vi "Pick or Place Part.vi"(5 "Part Vacuum Line":string, 6 "Pick or Place":enum16{"Pick", "Place"}(ring), 7 "Part Named Position":string, 8 "error in (no error)":errorcluster, 9 "Part Rotation":dbl, 10 "Part Position":refnum<class "Vec3d.lvclass">, 11 "Gantry in":refnum<class "Gantry.lvclass">) -> (0 "error out":errorcluster, 3 "Gantry out":refnum<class "Gantry.lvclass">)   [LabVIEW 2022 SP3, in "Gantry.lvclass"]
uses:
  Gantry.lvclass
  Vec3d Class/Vec3d.lvclass
  FlexWorktable/FlexWorktable.lvclass
  Gantry.lvclass/Gantry.ctl
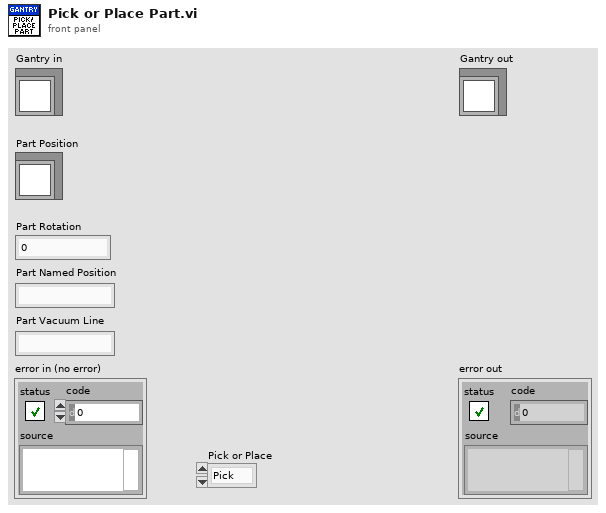
[diagram p1: front panel]
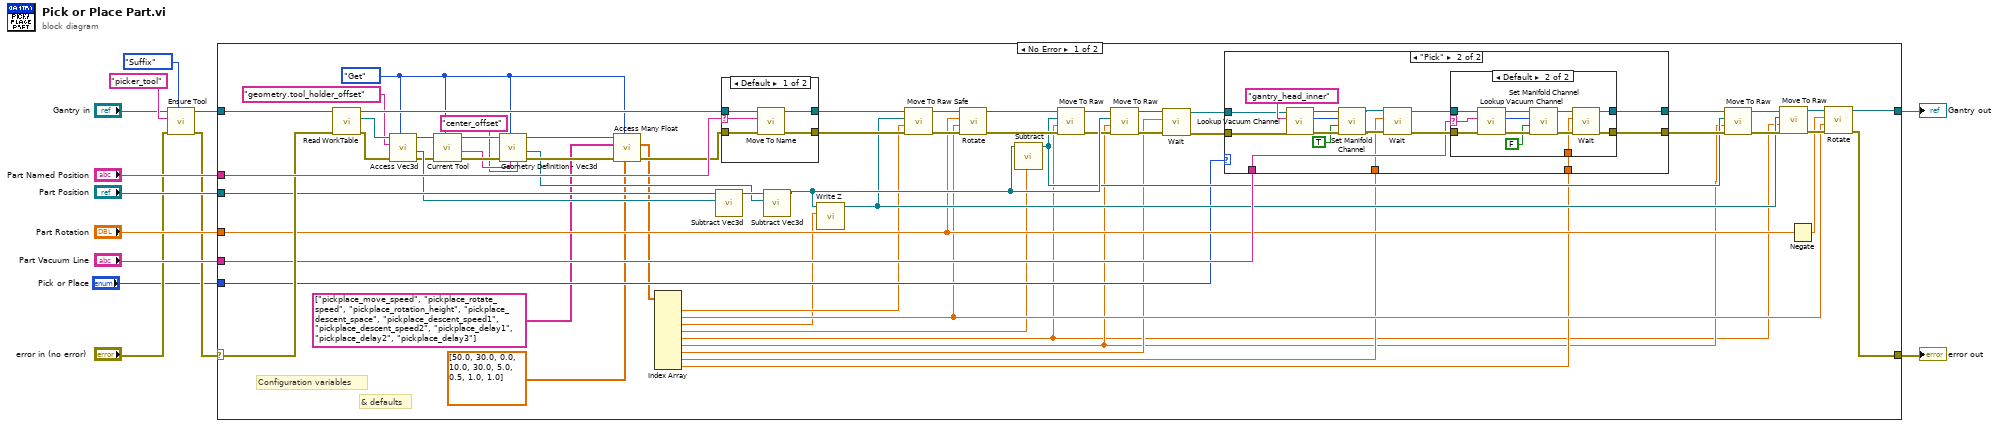
[diagram p0: block diagram]
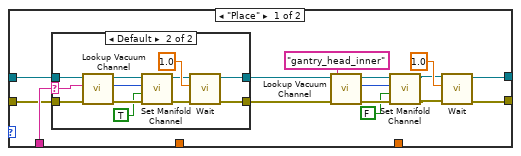
[diagram p2: hidden frame]
diagram:
  n1 = call "Ensure Tool.vi"("Match Type"=enum16{"Full", "Suffix"}."Suffix", "error in (no error)"="error in (no error)", "Tool Name"="picker_tool", "Gantry in"="Gantry in") -> ("error out"=w2:errorcluster, "Gantry out"=w4:refnum<class "Gantry.lvclass">)  [unwired: 6 in]
  n2 = case shown="No Error" w2 {
    selector: w2 -> [w68 w141]
    tunnel: [w32 w141] -> w13
    tunnel: [w33 w140] -> w12
    tunnel: w4 -> [w70 w140]
    tunnel: "Part Named Position" -> [w73 _]
    tunnel: "Part Position" -> [w64 _]
    tunnel: "Part Rotation" -> [w35 _]
    tunnel: "Part Vacuum Line" -> [w44 _]
    tunnel: "Pick or Place" -> [w31 _]
    frame No Error {
      w25 = enum16{"Get", "Set"}."Get" ("Get/Set")
      # "& defaults"
      # "Configuration variables"
      n3 = call-dynamic "Read WorkTable.vi"("error in"=w68, "Gantry Class in"=w70) -> ("error out"=w66:errorcluster, "Worktable"=w67:refnum<class "FlexWorktable.lvclass">, "Gantry Class out"=w69:refnum<class "Gantry.lvclass">)  [unwired: 7 in]
      n4 = call-dynamic "Access Vec3d.vi"("Get/Set"=w25, "error in (no error)"=w66, "Key"="geometry.tool_holder_offset", "FlexWorktable in"=w67) -> ("error out"=w60:errorcluster, "Value out"=w63:refnum<class "Vec3d.lvclass">, "FlexWorktable out"=w62:refnum<class "FlexWorktable.lvclass">)  [unwired: 5 in]
      n5 = call-dynamic "Current Tool.vi"("Get/Set"=w25, "error in (no error)"=w60, "FlexWorktable in"=w62) -> ("error out"=w59:errorcluster, "Tool out"=w58:string, "FlexWorktable out"=w61:refnum<class "FlexWorktable.lvclass">)  [unwired: 5 in, 1 out]
      n6 = call-dynamic "Geometry Definition - Vec3d.vi"("Feature Name"="center_offset", "Part Type"=w58, "Get/Set"=w25, "error in (no error)"=w59, "FlexWorktable in"=w61) -> ("error out"=w29:errorcluster, "Geometry Definition out"=w27:refnum<class "Vec3d.lvclass">, "FlexWorktable out"=w30:refnum<class "FlexWorktable.lvclass">)  [unwired: 4 in]
      n7 = call "Access Many Float.vi"("Defaults"=dbl[] [50.0, 30.0, 0.0, 10.0, 30.0, 5.0, 0.5, 1.0, 1.0], "Get/Set"=w25, "error in (no error)"=w29, "Keys"=string[] ["pickplace_move_speed", "pickplace_rotate_speed", "pickplace_rotation_height", "pickplace_descent_space", "pickplace_descent_speed1", "pickplace_descent_speed2", "pickplace_delay1", "pickplace_delay2", "pickplace_delay3"], "FlexWorktable in"=w30) -> ("error out"=w28:errorcluster, "Values out"=w23:dbl[])  [unwired: 4 in, 1 out]
      n8 = Index Array(array=w23) -> (element #1=w22:dbl, element #2=w21:dbl, element #3=w20:dbl, element #4=w19:dbl, element #5=w14:dbl, element #6=w15:dbl, element #7=w18:dbl, element #8=w17:dbl, element #9=w16:dbl)  [unwired: 9 in]
      n9 = call "Subtract Vec3d.vi"("Vec3d in 2"=w63, "Vec3d in 1"=w64) -> ("Vec3d Class out"=w56:refnum<class "Vec3d.lvclass">)  [unwired: 8 in, 1 out]
      n10 = case shown="Default" w73 {
        selector: w73 -> [w136 _]
        tunnel: w69 -> [w137 w139]
        tunnel: w28 -> [w135 w138]
        tunnel: [w134 w138] -> w71
        tunnel: [w133 w139] -> w72
        frame Default {
          n11 = call-dynamic "Move To Name.vi"("error in"=w135, "Destination"=w136, "Gantry in"=w137) -> ("error out"=w134:errorcluster, "Gantry out"=w133:refnum<class "Gantry.lvclass">)  [unwired: 6 in, 1 out]
        }
        frame "" {
        }
      }
      n12 = call "Subtract Vec3d.vi"("Vec3d in 2"=w27, "Vec3d in 1"=w56) -> ("Vec3d Class out"=w50:refnum<class "Vec3d.lvclass">)  [unwired: 8 in, 1 out]
      n13 = call-dynamic "Write Z.vi"("Z"=w20, "Vec3d Class in"=w50) -> ("Vec3d Class out"=w38:refnum<class "Vec3d.lvclass">)  [unwired: 8 in, 1 out]
      n14 = call-dynamic "Move To Raw Safe.vi"("error in"=w71, "Speed(mm/s)"=w22, "Destination"=w38, "Gantry in"=w72) -> ("error out"=w53:errorcluster, "Gantry out"=w55:refnum<class "Gantry.lvclass">)  [unwired: 6 in]
      n15 = call-dynamic "Rotate.vi"("error in"=w53, "speed(deg/s)"=w21, "distance(deg)"=w35, "Gantry in"=w55) -> ("error out"=w52:errorcluster, "Gantry out"=w54:refnum<class "Gantry.lvclass">)  [unwired: 6 in]
      n16 = call-dynamic "Subtract.vi"("Z"=w19, "Vec3d in"=w50) -> ("Vec3d  out"=w41:refnum<class "Vec3d.lvclass">)  [unwired: 8 in, 1 out]
      n17 = call-dynamic "Move To Raw.vi"("error in"=w52, "Speed"=w14, "Destination"=w41, "Gantry in"=w54) -> ("error out"=w49:errorcluster, "Gantry out"=w51:refnum<class "Gantry.lvclass">)  [unwired: 6 in]
      n18 = call-dynamic "Move To Raw.vi"("error in"=w49, "Speed"=w15, "Destination"=w50, "Gantry in"=w51) -> ("error out"=w47:errorcluster, "Gantry out"=w48:refnum<class "Gantry.lvclass">)  [unwired: 6 in]
      n19 = call "Wait.vi"("error in (no error)"=w47, "seconds"=w18, "Gantry in"=w48) -> ("error out"=w45:errorcluster, "Gantry out"=w46:refnum<class "Gantry.lvclass">)  [unwired: 7 in]
      n20 = case shown="\"Pick\"" w31 {
        tunnel: w46 -> [w88 w114]
        tunnel: w45 -> [w86 w113]
        tunnel: w44 -> [w87 w105]
        tunnel: [w77 w108] -> w43
        tunnel: [w76 w107] -> w42
        tunnel: w17 -> [_ w104]
        tunnel: w16 -> [_ w103]
        frame "Place" {
          n21 = case shown="Default" w87 {
            selector: w87 -> [_ w99]
            tunnel: w88 -> [w90 w98]
            tunnel: w86 -> [w89 w97]
            tunnel: [w90 w93] -> w78
            tunnel: [w89 w92] -> w75
            frame "" {
            }
            frame Default {
              n22 = call-dynamic "Lookup Vacuum Channel.vi"("error in (no error)"=w97, "Channel Name"=w99, "Gantry Class in"=w98) -> ("error out"=w101:errorcluster, "Channel Number"=w100:i32, "Gantry Class out"=w102:refnum<class "Gantry.lvclass">)  [unwired: 5 in]
              n23 = call-dynamic "Set Manifold Channel.vi"("error in"=w101, "On/Off"=TRUE, "Manifold Channel"=w100, "Gantry in"=w102) -> ("error out"=w94:errorcluster, "Gantry out"=w95:refnum<class "Gantry.lvclass">)  [unwired: 6 in]
              n24 = call "Wait.vi"("error in (no error)"=w94, "seconds"=1.0, "Gantry in"=w95) -> ("error out"=w92:errorcluster, "Gantry out"=w93:refnum<class "Gantry.lvclass">)  [unwired: 7 in]
            }
          }
          n25 = call-dynamic "Lookup Vacuum Channel.vi"("error in (no error)"=w75, "Channel Name"="gantry_head_inner", "Gantry Class in"=w78) -> ("error out"=w84:errorcluster, "Channel Number"=w83:i32, "Gantry Class out"=w85:refnum<class "Gantry.lvclass">)  [unwired: 5 in]
          n26 = call-dynamic "Set Manifold Channel.vi"("error in"=w84, "On/Off"=FALSE, "Manifold Channel"=w83, "Gantry in"=w85) -> ("error out"=w80:errorcluster, "Gantry out"=w81:refnum<class "Gantry.lvclass">)  [unwired: 6 in]
          n27 = call "Wait.vi"("error in (no error)"=w80, "seconds"=1.0, "Gantry in"=w81) -> ("error out"=w76:errorcluster, "Gantry out"=w77:refnum<class "Gantry.lvclass">)  [unwired: 7 in]
        }
        frame "Pick" {
          n28 = call-dynamic "Lookup Vacuum Channel.vi"("error in (no error)"=w113, "Channel Name"="gantry_head_inner", "Gantry Class in"=w114) -> ("error out"=w117:errorcluster, "Channel Number"=w116:i32, "Gantry Class out"=w118:refnum<class "Gantry.lvclass">)  [unwired: 5 in]
          n29 = call-dynamic "Set Manifold Channel.vi"("error in"=w117, "On/Off"=TRUE, "Manifold Channel"=w116, "Gantry in"=w118) -> ("error out"=w111:errorcluster, "Gantry out"=w112:refnum<class "Gantry.lvclass">)  [unwired: 6 in]
          n30 = call "Wait.vi"("error in (no error)"=w111, "seconds"=w104, "Gantry in"=w112) -> ("error out"=w109:errorcluster, "Gantry out"=w110:refnum<class "Gantry.lvclass">)  [unwired: 7 in]
          n31 = case shown="Default" w105 {
            selector: w105 -> [_ w129]
            tunnel: w110 -> [w120 w128]
            tunnel: w109 -> [w119 w127]
            tunnel: [w120 w124] -> w108
            tunnel: [w119 w123] -> w107
            tunnel: w103 -> [_ w121]
            frame "" {
            }
            frame Default {
              n32 = call-dynamic "Lookup Vacuum Channel.vi"("error in (no error)"=w127, "Channel Name"=w129, "Gantry Class in"=w128) -> ("error out"=w131:errorcluster, "Channel Number"=w130:i32, "Gantry Class out"=w132:refnum<class "Gantry.lvclass">)  [unwired: 5 in]
              n33 = call-dynamic "Set Manifold Channel.vi"("error in"=w131, "On/Off"=FALSE, "Manifold Channel"=w130, "Gantry in"=w132) -> ("error out"=w125:errorcluster, "Gantry out"=w126:refnum<class "Gantry.lvclass">)  [unwired: 6 in]
              n34 = call "Wait.vi"("error in (no error)"=w125, "seconds"=w121, "Gantry in"=w126) -> ("error out"=w123:errorcluster, "Gantry out"=w124:refnum<class "Gantry.lvclass">)  [unwired: 7 in]
            }
          }
        }
      }
      n35 = call-dynamic "Move To Raw.vi"("error in"=w42, "Speed"=w15, "Destination"=w41, "Gantry in"=w43) -> ("error out"=w39:errorcluster, "Gantry out"=w40:refnum<class "Gantry.lvclass">)  [unwired: 6 in]
      n36 = call-dynamic "Move To Raw.vi"("error in"=w39, "Speed"=w14, "Destination"=w38, "Gantry in"=w40) -> ("error out"=w36:errorcluster, "Gantry out"=w37:refnum<class "Gantry.lvclass">)  [unwired: 6 in]
      n37 = Negate(x=w35) -> (-x=w34:dbl)
      n38 = call-dynamic "Rotate.vi"("error in"=w36, "speed(deg/s)"=w21, "distance(deg)"=w34, "Gantry in"=w37) -> ("error out"=w32:errorcluster, "Gantry out"=w33:refnum<class "Gantry.lvclass">)  [unwired: 6 in]
    }
    frame Error {
    }
  }
  "error out" <- w13
  "Gantry out" <- w12
